vi "front wheel drive.vi"() -> ()   [LabVIEW 2009]
uses:
  <vilib>/NXT/Block Support/NXT_ButtonSelector.ctl
  <vilib>/NXT/Subs/MotorOutput.ctl
  <vilib>/NXT/Block Support/NXT_OutputPort.ctl
panel:
  out "period":u32
  out "integral":sgl format="%.2f"
  out "Error":i16
  out "drive mode":u8(ring) items=["Right"=1, "Left"=2, "Straight"=3]
  out "steer power output":sgl format="%.2f"
  out "steer PV":i16
  in  "Steering PID":cluster{"P":sgl, "I":sgl, "D":sgl}
  out "steer setpoint":i16
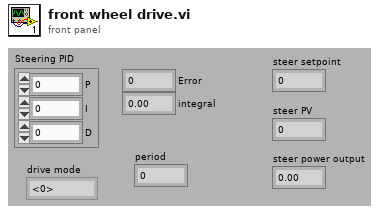
[diagram p1: front panel]
types:
  T1 = typedef "NXT_OutputPort.ctl" = u8
  T2 = typedef "MotorOutput.ctl" = u8
  T3 = typedef "NXT_ButtonSelector.ctl" = u16
  T4 = typedef "LVHSConnector.ctl" = cluster{"error":errorcluster, "address":string, "NXT #":i32, "Show Error":bool, "Connection":u16}
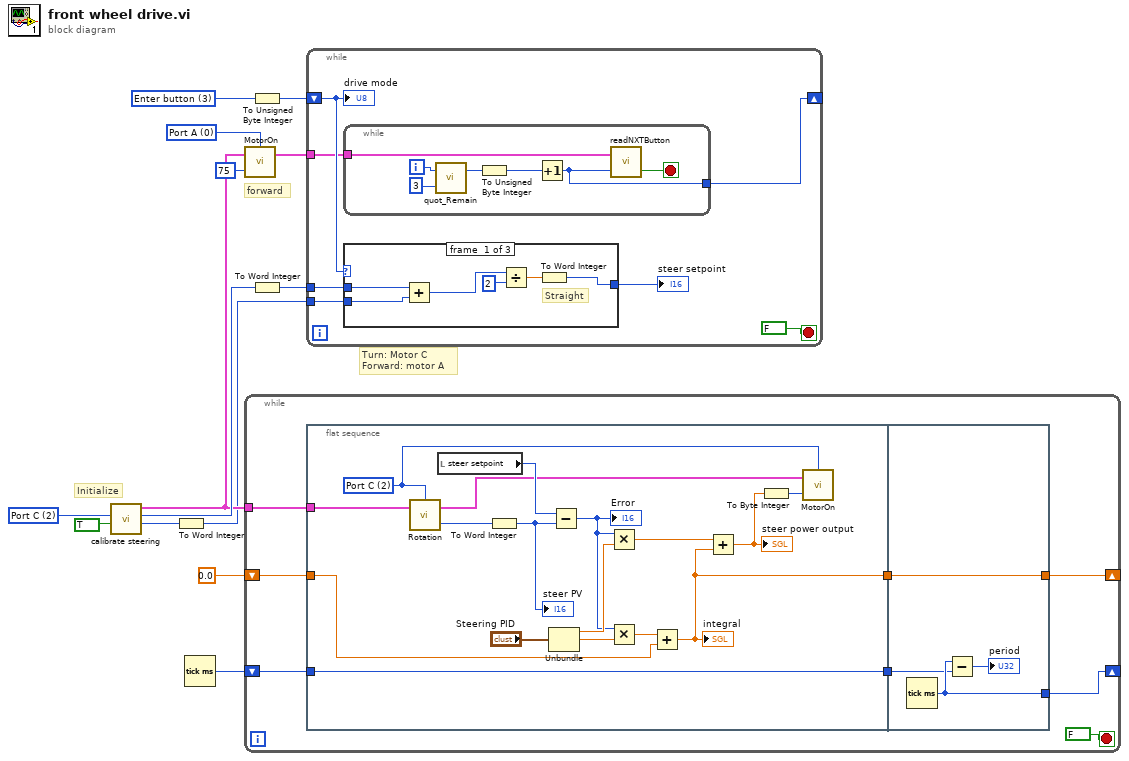
[diagram p0: block diagram]
diagram:
  w3 = T1 2 items=["Port A", "Port B", "Port C"] ("Steer motor port")
  w10 = T2 0 items=["Port A", "Port B", "Port C", "All Ports"] ("Output Port (All Ports)")
  w12 = T3 3 items=["Enter button"=3, "Left button"=2, "Right button"=1] ("Button (Enter button)")
  # "forward"
  # "Turn: Motor C\nForward: motor A"
  # "Initialize"
  n1 = call "calibrate steering.vi"("Flip direction?"=TRUE, "Steer motor port"=w3) -> ("Full right"=w13:i16, "Full left"=w14:i16, "NXT 2"=w9:T4)  [unwired: 7 in]
  n2 = To Word Integer(number=w13) -> (16bit integer=w6:i16)
  n3 = Tick Count (ms)() -> (millisecond timer value=w4:u32)
  n4 = call <vilib>:"MotorOn.vi"("Power (75)"=i8 75, "NXT"=w9, "Output Port (All Ports)"=w10) -> ("NXT"=w11:T4)  [unwired: 1 in]
  n5 = while {
    tunnel: w9 -> [w21]
    shift-right: [w19] -> _
    shift-left: sgl 0.0 -> [w20]
    shift-right: [w17] -> _
    shift-left: w4 -> [w15]
    stop <- FALSE stop-if-true
    n6 = flat-sequence {
      tunnel: w21 -> [w38]
      tunnel: w20 -> [w32]
      tunnel: [w26] -> w18
      tunnel: [w25] -> w16
      tunnel: w15 -> [w25]
      tunnel: [w43] -> w19
      tunnel: w18 -> [w43]
      tunnel: [w42] -> w17
      tunnel: w16 -> [w41]
      frame #0 {
        w24 = T1 2 items=["Port A", "Port B", "Port C"] ("Port (Port A)")
        n7 = call <vilib>:"Rotation.vi"("NXT"=w38, "Port (Port A)"=w24) -> ("Rotation"=w37:i32, "NXT"=w28:T4)  [unwired: 1 in]
        n8 = local read "steer setpoint"() -> (w39:i16)
        n9 = To Word Integer(number=w37) -> (16bit integer=w33:i16)
        "steer PV" <- w33
        n10 = Unbundle("Steering PID") -> ("P"=w35:sgl, "I"=w31:sgl)  [unwired: 1 out]
        n11 = Subtract(x=w39, y=w33) -> (x-y=w34:i16)
        "Error" <- w34
        n12 = Multiply(x=w34, y=w35) -> (x*y=w29:sgl)
        n13 = Multiply(x=w34, y=w31) -> (x*y=w30:sgl)
        n14 = Add(x=w30, y=w32) -> (x+y=w26:sgl)
        "integral" <- w26
        n15 = Add(x=w29, y=w26) -> (x+y=w27:sgl)
        "steer power output" <- w27
        n16 = To Byte Integer(number=w27) -> (8bit integer=w23:i8)
        n17 = call <vilib>:"MotorOn.vi"("Power (75)"=w23, "NXT"=w28, "Output Port (All Ports)"=w24) -> ()  [unwired: 1 in, 1 out]
      }
      frame #1 {
        n18 = Tick Count (ms)() -> (millisecond timer value=w42:u32)
        n19 = Subtract(x=w42, y=w41) -> (x-y=→"period":u32)
      }
    }
  }
  n20 = To Unsigned Byte Integer(number=w12) -> (unsigned 8bit integer=w8:u8)
  n21 = To Word Integer(number=w14) -> (16bit integer=w7:i16)
  n22 = while {
    shift-right: [w48] -> _
    shift-left: w8 -> [w50]
    tunnel: w7 -> [w47]
    tunnel: w6 -> [w46]
    tunnel: w11 -> [w44]
    stop <- FALSE stop-if-true
    n23 = while {
      tunnel: [w52] -> w48
      tunnel: w44 -> [w53]
      i -> [w57]
      stop <- w54 stop-if-true
      n24 = call <vilib>:"quot_Remain.vi"("y"=3, "x"=w57) -> ("x-y*floor(x/y)"=w55:i32)  [unwired: 1 out]
      n25 = To Unsigned Byte Integer(number=w55) -> (unsigned 8bit integer=w51:u8)
      n26 = Increment(x=w51) -> (x+1=w52:u8)
      n27 = call <vilib>:"readNXTButton.vi"("Button (Enter button)"=w52, "NXT"=w53) -> ("Yes/No"=w54:bool)  [unwired: 1 in, 1 out]
    }
    n28 = case shown="3, Default" w50 {
      tunnel: w47 -> [w63 _ w65]
      tunnel: w46 -> [w62 w64 _]
      tunnel: [w58 w64 w65] -> w45
      frame #0 {
        # "Straight"
        n29 = Add(x=w63, y=w62) -> (x+y=w61:i16)
        n30 = Divide(x=w61, y=i16 2) -> (x/y=w59:dbl)
        n31 = To Word Integer(number=w59) -> (16bit integer=w58:i16)
      }
      frame #1 {
        # "Right"
      }
      frame #2 {
        # "Left"
      }
    }
    "steer setpoint" <- w45
    "drive mode" <- w50
  }
